vi "Get Transfer Identifier from Map.vi"(7 "Transfer ID map":map{u32, u32}(c390), 8 "error in":errorcluster, 9 "label information":cluster{"label number":T1, "sdi":u8} {"label number" format="%.0o"}, 10 "channel number in":u8, 11 "board number in":u8) -> (0 "error out":errorcluster, 3 "Transfer ID out":u32)   [LabVIEW 2024, in "AIM ARINC 429 Hardware API.lvlib"]
uses:
  AIM ARINC 429 Hardware API.lvlib
  Shared/Label.ctl
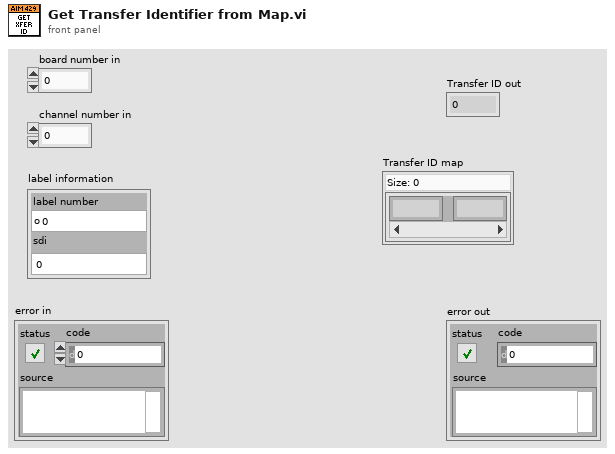
[diagram p1: front panel]
types:
  T1 = typedef "Label.ctl" = u8
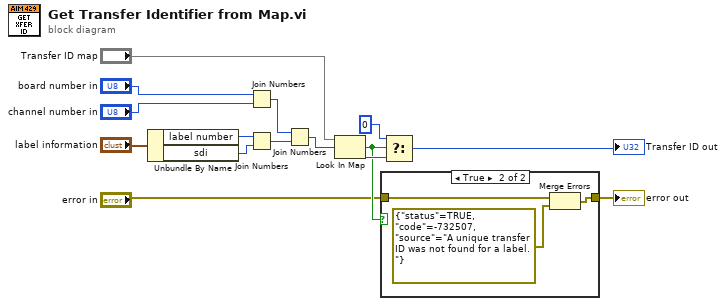
[diagram p0: block diagram]
diagram:
  n1 = Unbundle By Name("label information") -> ("label number"=w12:T1, "sdi"=w11:u8)
  n2 = Join Numbers(hi="board number in", lo="channel number in") -> ((hi.lo)=w10:u16)
  n3 = Join Numbers(hi=w12, lo=w11) -> ((hi.lo)=w9:u16)
  n4 = Join Numbers(hi=w10, lo=w9) -> ((hi.lo)=w8:u32)
  n5 = Look In Map(map="Transfer ID map", key=w8) -> (key not found?=w3:bool, value=w4:u32)  [unwired: 1 in]
  n6 = case shown="True" w3 {
    tunnel: "error in" -> [w16 w19]
    tunnel: [w16 w17] -> w1
    frame False {
    }
    frame True {
      n7 = Merge Errors(w19, errorcluster {"status"=TRUE, "code"=-732507, "source"="A unique transfer ID was not found for a label."} ("error constant")) -> (w17:errorcluster)
    }
  }
  "error out" <- w1
  n8 = Select(t=u32 0 ("value"), s=w3, f=w4) -> (s? t:f=→"Transfer ID out":u32)
